vi "Initialize.vi"(8 "error in (no error)":errorcluster, 11 "GRMActor in":refnum<class "FlatField.lvclass">) -> (0 "error out":errorcluster, 3 "GRMActor out":refnum<class "FlatField.lvclass">)   [LabVIEW 2020, in "FlatField.lvlib" / "FlatField.lvclass"]
uses:
  FlatField.lvclass
  FlatField Status.ctl
  Displayer/Displayer/FlatField Method.ctl
  FlatField.lvclass/FlatField.ctl
  Hardware Abstraction Layer/Component/GenericActor/GenericActor/GenericController.lvclass
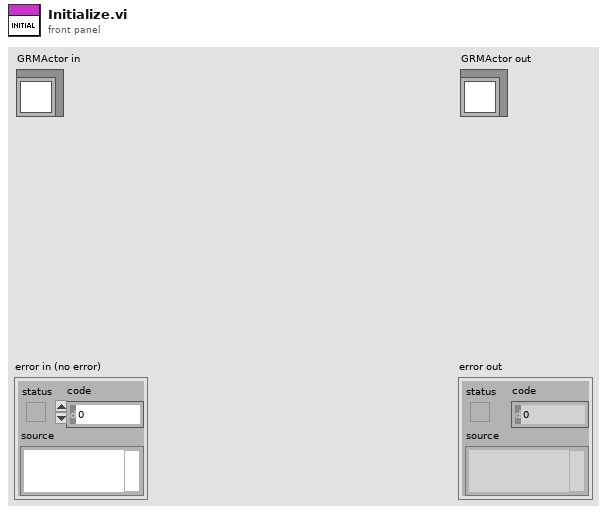
[diagram p1: front panel]
types:
  T1 = typedef "FlatField.lvlib/FlatField.lvclass/FlatField Method.ctl" = i32
  T2 = typedef "Image Type" = u32
  T3 = typedef "FlatField.lvlib/FlatField.lvclass/FlatField Status.ctl" = i32
  T4 = typedef "IMAQ Image.ctl" = refnum<image>
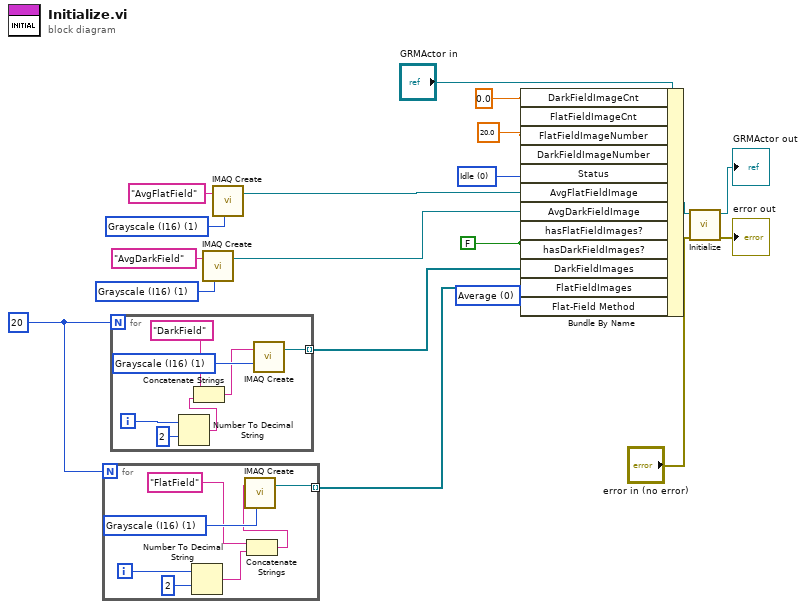
[diagram p0: block diagram]
diagram:
  w1 = T1 0 items=["Average", "Median"] ("Flat-Field Method")
  w4 = 20
  w5 = FALSE ("hasFlatFieldImages?")
  w8 = T2 1 items=["Grayscale (U8)", "Grayscale (I16)", "Grayscale (SGL)", "Complex (CSG)", "RGB (U32)", "HSL (U32)", "RGB (U64)", "Grayscale (U16)"] ("Image Type")
  w9 = T2 1 items=["Grayscale (U8)", "Grayscale (I16)", "Grayscale (SGL)", "Complex (CSG)", "RGB (U32)", "HSL (U32)", "RGB (U64)", "Grayscale (U16)"] ("Image Type")
  w12 = 0.0 ("DarkFieldImageCnt")
  w13 = 20.0 ("FieldFieldImageNumber")
  w14 = T3 0 items=["Idle", "Taking DarkField Images", "Taking FlatField Image", "Doing FlatField", ""] ("Flat-Field Status")
  n1 = for {
    N: w4 -> [_]
    tunnel: [w20] -> w2 mode=indexing
    i -> [w25]
    w26 = T2 1 items=["Grayscale (U8)", "Grayscale (I16)", "Grayscale (SGL)", "Complex (CSG)", "RGB (U32)", "HSL (U32)", "RGB (U64)", "Grayscale (U16)"] ("Image Type")
    n2 = Number To Decimal String(number=w25, width (-)=i16 2) -> (decimal integer string=w22:string)
    n3 = Concatenate Strings("FlatField" ("Image Name"), w22) -> (w21:string)
    n4 = call "IMAQ Create"("Image Name"=w21, "Image Type"=w26) -> ("New Image"=w20:T4)  [unwired: 3 in, 1 out]
  }
  n5 = for {
    N: w4 -> [_]
    tunnel: [w27] -> w3 mode=indexing
    i -> [w32]
    w33 = T2 1 items=["Grayscale (U8)", "Grayscale (I16)", "Grayscale (SGL)", "Complex (CSG)", "RGB (U32)", "HSL (U32)", "RGB (U64)", "Grayscale (U16)"] ("Image Type")
    n6 = Number To Decimal String(number=w32, width (-)=i16 2) -> (decimal integer string=w30:string)
    n7 = Concatenate Strings("DarkField" ("Image Name"), w30) -> (w28:string)
    n8 = call "IMAQ Create"("Image Name"=w28, "Image Type"=w33) -> ("New Image"=w27:T4)  [unwired: 3 in, 1 out]
  }
  n9 = call "IMAQ Create"("Image Name"="AvgDarkField", "Image Type"=w8) -> ("New Image"=w6:T4)  [unwired: 3 in, 1 out]
  n10 = call "IMAQ Create"("Image Name"="AvgFlatField", "Image Type"=w9) -> ("New Image"=w11:T4)  [unwired: 3 in, 1 out]
  n11 = Bundle By Name(cluster="GRMActor in", "DarkFieldImageCnt"=w12, "FlatFieldImageCnt"=w12, "FlatFieldImageNumber"=w13, "DarkFieldImageNumber"=w13, "Status"=w14, "AvgFlatFieldImage"=w11, "AvgDarkFieldImage"=w6, "hasFlatFieldImages?"=w5, "hasDarkFieldImages?"=w5, "DarkFieldImages"=w3, "FlatFieldImages"=w2, "Flat-Field Method"=w1) -> (w15:refnum<class "FlatField.lvclass">)
  n12 = call-parent "Initialize.vi"("error in (no error)"="error in (no error)", "GRMActor in"=w15) -> ("error out"=→"error out":errorcluster, "GRMActor out"=→"GRMActor out":refnum<class "FlatField.lvclass">)  [unwired: 8 in]
